vi "List Certificates.vi"(8 "error in (no error)":errorcluster, 11 "IoT Session in":refnum<class "IoT Session.lvclass">) -> (0 "error out":errorcluster, 2 "Certificate IDs":string[](array[string]), 3 "IoT Session out":refnum<class "IoT Session.lvclass">)   [LabVIEW 2015, in "NI_AWS_IoT.lvlib" / "IoT Session.lvclass"]
uses:
  IoT Session.lvclass
  Core/HTTP Request/Request Options.ctl
  Core/HTTP Request/Name Value Pair.ctl
  Core/HTTP Request/Region handling.ctl
  Core/HTTP Request/URL formatting.ctl
  Core/HTTP Request/HTTP Request.lvclass
  JSON Parsing/NI_JSON Parsing.lvlib
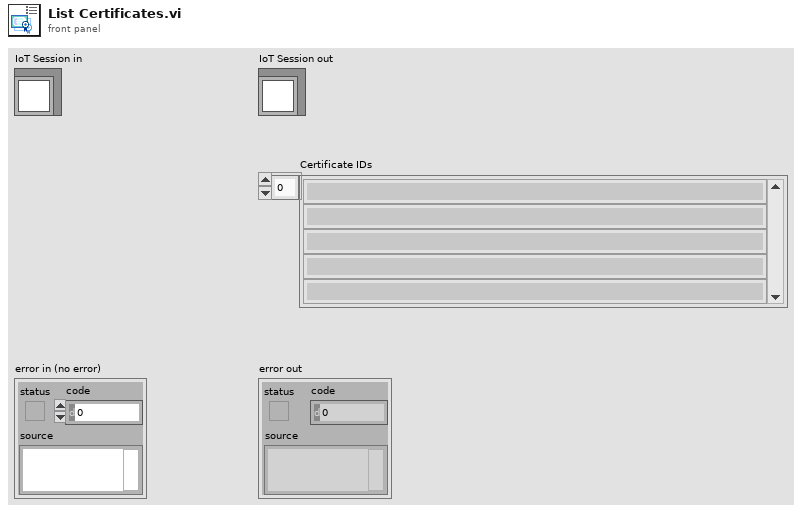
[diagram p1: front panel]
types:
  T1 = typedef "NI_AWS_Core.lvlib/HTTP Request.lvclass/Name Value Pair.ctl" = cluster{"name":string, "value":string}
  T2 = typedef "NI_AWS_Core.lvlib/HTTP Request.lvclass/Request Options.ctl" = cluster{"request headers":T1[], "request parameters":T1[], "request body":string, "region handling":T3, "URL formatting":T4}
  T3 = typedef "NI_AWS_Core.lvlib/HTTP Request.lvclass/Region handling.ctl" = enum16{"use region everywhere", "use region (authentication only)", "use region (URL only)", "ignore region everwhere"}
  T4 = typedef "NI_AWS_Core.lvlib/HTTP Request.lvclass/URL formatting.ctl" = enum16{"region-", "region."}
  T5 = typedef "NI_AWS_Core.lvlib/HTTP Request.lvclass/Response.ctl" = cluster{"Headers":string, "Body":string}
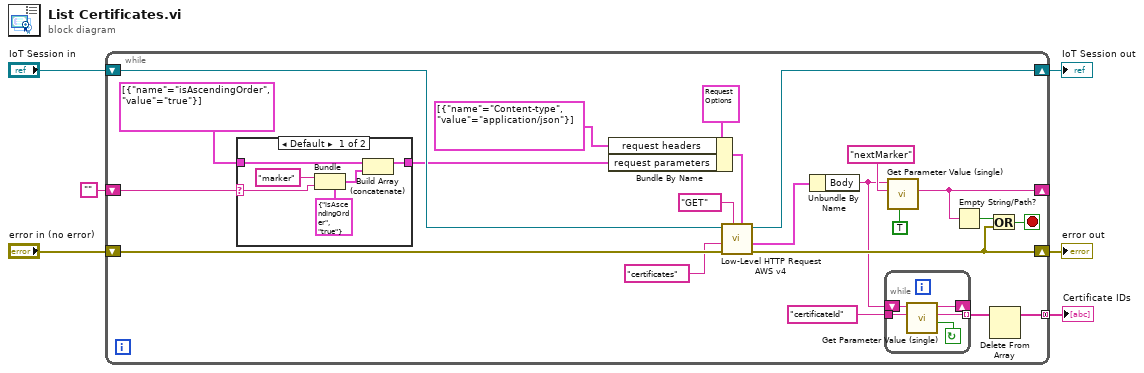
[diagram p0: block diagram]
diagram:
  n1 = while {
    shift-right: [w17] -> w5
    shift-left: "error in (no error)" -> [w25]
    shift-right: [w24] -> w4
    shift-left: "IoT Session in" -> [w23]
    shift-right: [w19] -> _
    shift-left: "" -> [w21]
    tunnel: [w7] -> w1 mode=concatenating
    stop <- w16 stop-if-true
    n2 = case shown="Default" w21 {
      selector: w21 -> [w30 _]
      tunnel: T1[] [{"name"="isAscendingOrder", "value"="true"}] ("request parameters") -> [w34 w35]
      tunnel: [w33 w35] -> w11
      frame Default {
        n3 = Bundle(cluster=T1 {"name"="isAscendingOrder", "value"="true"} ("Name Value Pair"), "name"="marker", "value"=w30) -> (w31:T1)
        n4 = Build Array (concatenate)(w34, w31) -> (w33:T1[])
      }
      frame "" {
      }
    }
    n5 = Bundle By Name(cluster=T2 {"request headers"=[], "request parameters"=[], "request body"="", "region handling"=enum."use region everywhere", "URL formatting"=enum."region."} ("Request Options"), "request headers"=T1[] [{"name"="Content-type", "value"="application/json"}], "request parameters"=w11) -> (w26:T2)
    n6 = call "Low-Level HTTP Request AWS v4.vi"("Request Options"=w26, "HTTP-Verb"="GET", "error in (no error)"=w25, "URL Suffix"="certificates" ("string"), "AWS Core in"=w23) -> ("error out"=w17:errorcluster, "Response"=w22:T5, "AWS Core out"=w24:refnum<class "IoT Session.lvclass">)  [unwired: 3 in, 1 out]
    n7 = Unbundle By Name(w22) -> ("Body"=w9:string)
    n8 = while {
      tunnel: "certificateId" ("Parameter Name") -> [w40]
      tunnel: [w39] -> w8 mode=indexing
      shift-right: [w37] -> _
      shift-left: w9 -> [w38]
      stop <- w36 continue-if-true
      n9 = call "Get Parameter Value (single).vi"("Parameter Name"=w40, "JSON"=w38) -> ("Found"=w36:bool, "Parameter Value"=w39:string, "Remaining JSON"=w37:string)  [unwired: 6 in, 1 out]
    }
    n10 = call "Get Parameter Value (single).vi"("Clear Null"=TRUE, "Parameter Name"="nextMarker", "JSON"=w9) -> ("Parameter Value"=w19:string)  [unwired: 5 in, 3 out]
    n11 = Empty String/Path?(string/path=w19) -> (empty?=w18:bool)
    n12 = Or(x=w18, y=w17) -> (x .or. y?=w16:bool)
    n13 = Delete From Array(array=w8) -> (array with subset deleted=w7:string[])  [unwired: 2 in, 1 out]
  }
  "error out" <- w5
  "IoT Session out" <- w4
  "Certificate IDs" <- w1
